vi "control disabler.vi"(8 "error in (no error)":errorcluster, 10 "Disabled":T1(ring), 11 "Array":refnum<vi>[](array[refnum])) -> (0 "error out":errorcluster)   [LabVIEW 2015]
doc: "Enables or disables control on front panel."
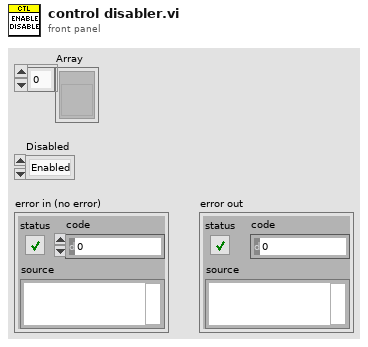
[diagram p1: front panel]
types:
  T1 = enum8{"Enabled", "Disabled", "Disabled and Grayed Out"}
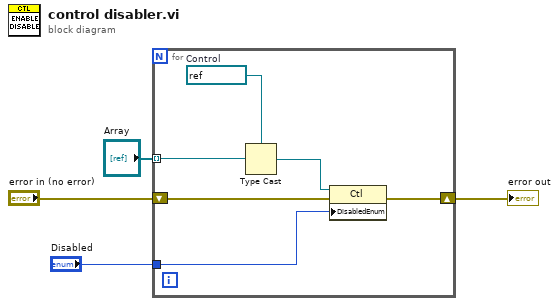
[diagram p0: block diagram]
diagram:
  n1 = for {
    tunnel: "Disabled" -> [w8]
    tunnel: "Array" -> [w5] mode=indexing
    shift-right: [w10] -> w4
    shift-left: "error in (no error)" -> [w9]
    w6 = refnum<vi> refnum  # Control
    n2 = Type Cast(type=w6, x=w5) -> (*(type *) &x=w7:refnum<vi>)
    n3 = property class="Ctl"(reference=w7, error in=w9, "DisabledEnum"=w8) -> (error out=w10:errorcluster)  [unwired: 1 out]
  }
  "error out" <- w4
